vi "Arduino Blinky.vi"() -> ()   [LabVIEW 2020]
uses:
  <vilib>/MakerHub/LINX/Public/Peripherals/Digital/Digital Write 1 Chan.vi
  <vilib>/MakerHub/LINX/Public/Peripherals/Digital/Digital Write N Chans.vi
  <vilib>/MakerHub/LINX/Private/Local IO/LinxDigitalWrite.vi
  <vilib>/MakerHub/LINX/Public/Utilities/Check Channel.vi
  <vilib>/MakerHub/LINX/Public/Utilities/Open Serial.vi
  <vilib>/MakerHub/LINX/Private/Utilties/Generate Error.vi
  <vilib>/MakerHub/LINX/LMH-LINX.lvlib
panel:
  in  "stop":bool
  out "LED":bool
  out "Device Name":string
  in  "milliseconds to wait":u32
  out "Error Out":errorcluster
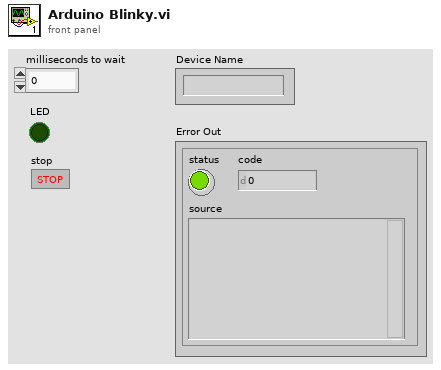
[diagram p1: front panel]
types:
  T1 = typedef "LMH-LINX.lvlib/LINX Ref.ctl" = cluster{"IO":T2, "Interface":T3, "LINX Device Config":T4}
  T2 = typedef "LMH-LINX.lvlib/Platform.ctl" = enum16{"Remote", "Local"}
  T3 = typedef "LMH-LINX.lvlib/Interface.ctl" = enum16{"Serial", "TCP"}
  T4 = typedef "LMH-LINX.lvlib/Device.lvlib/LINX Device Config.ctl" = cluster{"Interface":T3, "COM Port":refnum<visa-resource-name>, "TCP Configuration":T5, "Device Family":u8, "Device ID":u8, "Device Name":string, "TCP Ref":refnum<k5>, "Channels":T6}
  T5 = typedef "LMH-LINX.lvlib/Device.lvlib/TCP Config.ctl" = cluster{"IP Address":string, "Port":u16}
  T6 = typedef "LMH-LINX.lvlib/Channels.ctl" = cluster{"DI":u8[], "DO":u8[], "AI":u8[], "AO":u8[], "PWM":u8[], "QE":u8[], "UART":u8[], "I2C 2":u8[], "SPI":u8[], "CAN":u8[], "Servo":u8[], "AI Ref (V)":dbl, "AI Resolution (Bits)":u8, "AO Ref (V)":dbl, "AO Resolution (Bits)":u8}
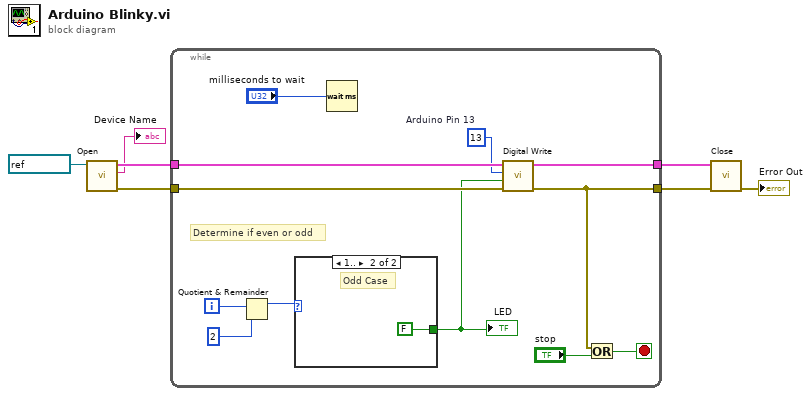
[diagram p0: block diagram]
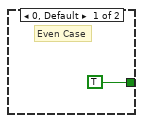
[diagram p2: hidden frame]
diagram:
  n1 = call-poly <vilib>:"Open.vi"("Serial Port"=refnum<visa-resource-name> "COM4") -> ("Error Out"=w2:errorcluster, "Device Name"=→"Device Name":string, "LINX Resource"=w4:T1)  [unwired: 8 in]
  n2 = while {
    tunnel: [w19] -> w5
    tunnel: w4 -> [w18]
    tunnel: [w9] -> w3
    tunnel: w2 -> [w16]
    i -> [w14]
    stop <- w11 stop-if-true
    w17 = u8 13  # Arduino Pin 13
    # "Determine if even or odd"
    n3 = Quotient & Remainder(x=w14, y=2) -> (x-y*floor(x/y)=w12:i32)  [unwired: 1 out]
    n4 = case shown="1.." w12 {
      tunnel: [TRUE FALSE] -> w8
      frame 0, Default {
        # "Even Case"
      }
      frame 1.. {
        # "Odd Case"
      }
    }
    "LED" <- w8
    n5 = Wait (ms)(milliseconds to wait="milliseconds to wait") -> ()  [unwired: 1 out]
    n6 = call-poly <vilib>:"Digital Write.vi"("Error In"=w16, "Output Value"=w8, "DO Channel"=w17, "LINX Resource"=w18) -> ("Error Out"=w9:errorcluster, "LINX Resource"=w19:T1)  [unwired: 6 in]
    n7 = Or(x=w9, y="stop") -> (x .or. y?=w11:bool)
  }
  n8 = call <vilib>:"Close.vi"("Error In"=w3, "LINX Resource"=w5) -> ("Error Out"=→"Error Out":errorcluster)  [unwired: 9 in]
